vi "Interpolate Values.vi"(6 "Digital":bool, 7 "Prioritize reaching values":bool, 8 "Values":dbl[](array[numeric]), 9 "Remaining Time":dbl, 10 "Time in Step":dbl, 11 "Duration":dbl) -> (3 "Value Out":dbl)   [LabVIEW 2020, in "Output Sequencer.lvlib" / "Output Sequencer.lvclass"]
uses:
  Output Sequencer.lvclass
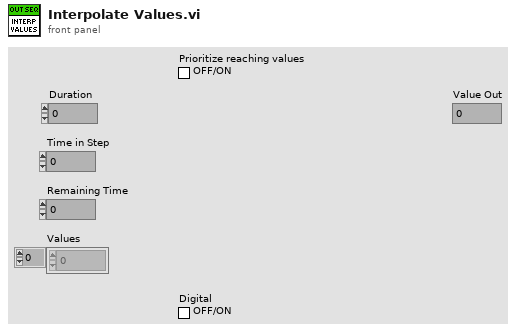
[diagram p1: front panel]
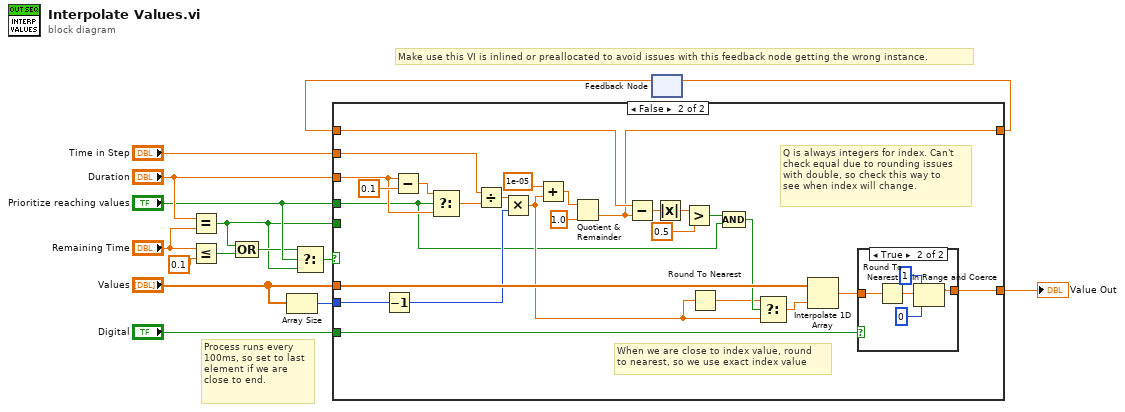
[diagram p0: block diagram]
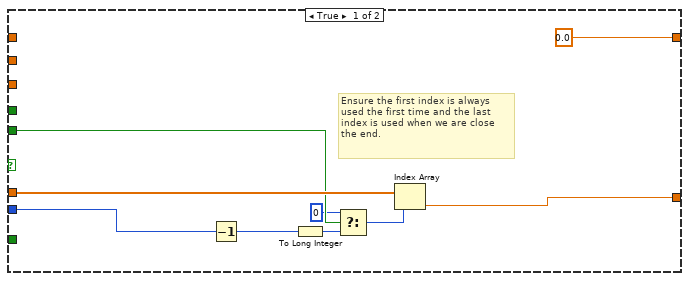
[diagram p2: hidden frame]
diagram:
  # "Make use this VI is inlined or preallocated to avoid issues with this feedback node getting the wrong instance."
  # "Process runs every 100ms, so set to last element if we are close to end."
  n1 = Equal?(x="Duration", y="Remaining Time") -> (x = y?=w1:bool)
  n2 = Less Or Equal?(x="Remaining Time", y=0.1) -> (x <= y?=w8:bool)
  n3 = Compound Arithmetic op=OR(w1, w8) -> (w4:bool)
  n4 = Array Size(array="Values") -> (size(s)=w9:i32)
  n5 = Select(t=w4, s="Prioritize reaching values", f=w1) -> (s? t:f=w3:bool)
  n6 = feedback #1() -> (w6:dbl)  [unwired: 1 in]
  n7 = case shown="False" w3 {
    tunnel: "Values" -> [w24 w50]
    tunnel: w9 -> [w18 w48]
    tunnel: "Duration" -> [_ w30]
    tunnel: "Time in Step" -> [_ w46]
    tunnel: [w21 w43] -> w12
    tunnel: w1 -> [w23 _]
    tunnel: "Digital" -> [_ w45]
    tunnel: [0.0 w39] -> w7
    tunnel: w6 -> [_ w40]
    tunnel: "Prioritize reaching values" -> [_ w27]
    frame True {
      # "Ensure the first index is always used the first time and the last index is used when we are close the end."
      n8 = Decrement(x=w18) -> (x-1=w17:i32)
      n9 = To Long Integer(number=w17) -> (32bit integer=w19:i32)
      n10 = Select(t=0 ("f"), s=w23, f=w19) -> (s? t:f=w22:i32)
      n11 = Index Array(array=w24, index=w22) -> (element=w21:dbl)
    }
    frame False {
      # "Q is always integers for index. Can't\ncheck equal due to rounding issues\nwith double, so check this way to\nsee when index will change."
      # "When we are close to index value, round\nto nearest, so we use exact index value"
      n12 = Decrement(x=w48) -> (x-1=w47:i32)
      n13 = Subtract(x=w30, y=0.1) -> (x-y=w32:dbl)
      n14 = Select(t=w32, s=w27, f=w30) -> (s? t:f=w29:dbl)
      n15 = Divide(x=w46, y=w29) -> (x/y=w49:dbl)
      n16 = Multiply(x=w49, y=w47) -> (x*y=w35:dbl)
      n17 = Add(x=1e-05, y=w35) -> (x+y=w33:dbl)
      n18 = Quotient & Remainder(x=w33, y=1.0) -> (floor(x/y)=w39:dbl)  [unwired: 1 out]
      n19 = Subtract(x=w40, y=w39) -> (x-y=w38:dbl)
      n20 = Absolute Value(x=w38) -> (abs(x)=w37:dbl)
      n21 = Greater?(x=w37, y=0.5) -> (0:w28:bool)
      n22 = Round To Nearest(number=w35) -> (nearest integer value=w25:dbl)
      n23 = Compound Arithmetic op=AND(w28, w27) -> (w26:bool)
      n24 = Select(t=w25, s=w26, f=w35) -> (s? t:f=w41:dbl)
      n25 = Interpolate 1D Array(1:w41, 2:w50) -> (0:w44:dbl)
      n26 = case shown="True" w45 {
        tunnel: w44 -> [w51 w56]
        tunnel: [w51 w54] -> w43
        frame False {
        }
        frame True {
          n27 = Round To Nearest(number=w56) -> (nearest integer value=w55:dbl)
          n28 = In Range and Coerce(upper limit=1, x=w55, lower limit=0) -> (coerced(x)=w54:dbl)  [unwired: 1 out]
        }
      }
    }
  }
  "Value Out" <- w12
  n29 = feedback-in #1(w7) -> ()
